vi "FileGetInfo.vi"(8 "error in (no error)":errorcluster, 10 "(Empty=No Action)":string caption="File Name", 11 "controller in":refnum<k24>) -> (0 "error out":errorcluster, 1 "File info Cluster":T1, 3 "controller out":refnum<k24>)   [LabVIEW 2019]
uses:
  C:/Users/patrick/Documents/GitHub/Aerotech-Delay-Line/lvsrc/Aerotech-Ensemble-LabVIEW/2010-5.6/Bin/Aerotech.Ensemble.dll
  Bin/Aerotech.Ensemble.dll
  C:/Users/patrick/Documents/GitHub/Aerotech-Delay-Line/lvsrc/Aerotech-Ensemble-LabVIEW/2010-5.6/Bin/Aerotech.Ensemble.LabVIEW.dll
  Bin/Aerotech.Ensemble.LabVIEW.dll
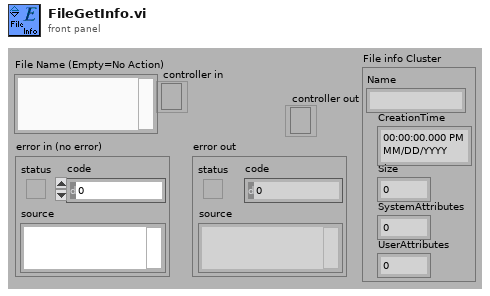
[diagram p1: front panel]
types:
  T1 = cluster{"Name":string, "CreationTime":timestamp, "Size":i32, "SystemAttributes":i32, "UserAttributes":i32}
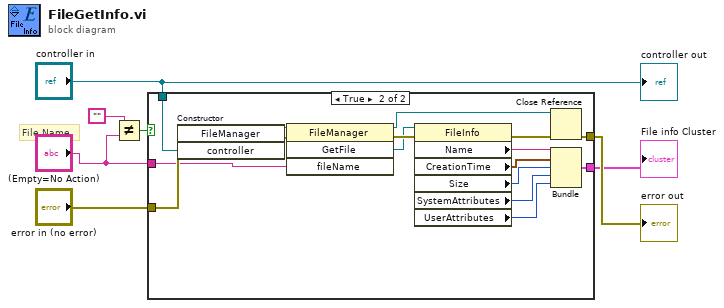
[diagram p0: block diagram]
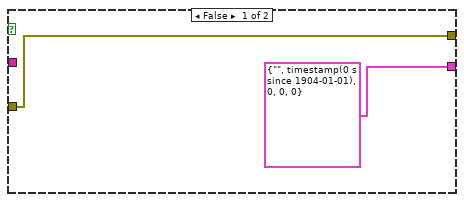
[diagram p2: hidden frame]
diagram:
  # "File Name"
  n1 = Not Equal?(x="", y="(Empty=No Action)") -> (x != y?=w3:bool)
  n2 = case shown="True" w3 {
    tunnel: [w9 w24] -> w7
    tunnel: "(Empty=No Action)" -> [_ w10]
    tunnel: "controller in" -> [_ w23]
    tunnel: "error in (no error)" -> [w9 w22]
    tunnel: [T1 {"Name"="", "CreationTime"=timestamp(0 s since 1904-01-01), "Size"=0, "SystemAttributes"=0, "UserAttributes"=0} w12] -> w4
    frame False {
    }
    frame True {
      n3 = constructor class="FileManager"(error in=w22, "controller"=w23) -> (reference out=w21:refnum<k24>, error out=w20:errorcluster)  [unwired: 2 in, 2 out]
      n4 = invoke class="FileManager" method="GetFile"(reference=w21, error in=w20, "fileName"=w10) -> (reference out=w25:refnum<k24>, error out=w19:errorcluster, "GetFile"=w11:refnum<k24>)  [unwired: 1 in, 1 out]
      n5 = property class="FileInfo"(reference=w11, error in=w19) -> (error out=w18:errorcluster, "Name"=w17:string, "CreationTime"=w16:timestamp, "Size"=w15:i32, "SystemAttributes"=w14:i32, "UserAttributes"=w13:i32)  [unwired: 1 out]
      n6 = Close Reference(reference=w25, error in (no error)=w18) -> (error out=w24:errorcluster)
      n7 = Bundle("Name"=w17, "CreationTime"=w16, "Size"=w15, "SystemAttributes"=w14, "UserAttributes"=w13) -> (w12:T1)  [unwired: 1 in]
    }
  }
  "error out" <- w7
  "File info Cluster" <- w4
  "controller out" <- "controller in"
